vi "GetUserLayouts.vi"(8 "error in (no error)":errorcluster, 11 "Layout Ring Refnum":refnum<vi>) -> (0 "error out":errorcluster, 1 "Non-user Strings And Values []":T1, 2 "Value":i32, 3 "User StringsAndValues[]":T1, 4 "Num User Layouts":i32)   [LabVIEW 2013]
doc: "SetList table layouts consist of \"default\" layouts (ring val < 0) and user layouts (ring val >0). This VI separates the two, returning the input ring's \"Value\", \"User Strings and Values[]\" and \"Non-user layouts\" (also StringAndValue array)."
uses:
  <vilib>/Utility/miscctls.llb/LVStringsAndValuesArrayTypeDef_I32.ctl
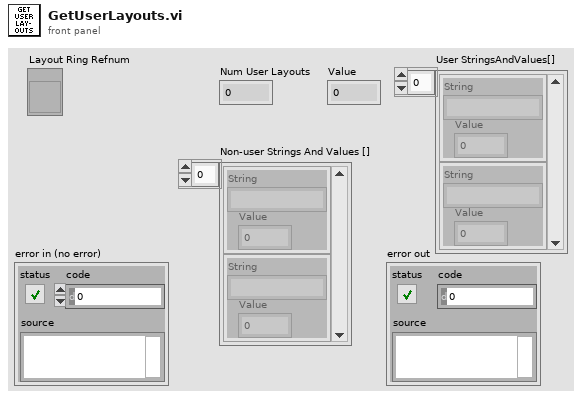
[diagram p1: front panel]
types:
  T1 = typedef "LVStringsAndValuesArrayTypeDef_I32.ctl" = cluster{"String":string, "Value":i32}[]
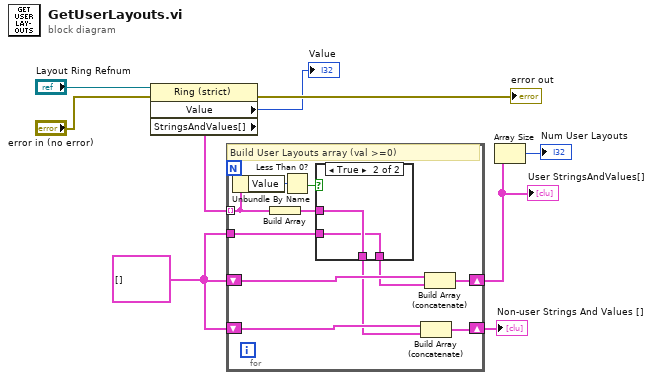
[diagram p0: block diagram]
diagram:
  w1 = T1 [] ("StringsAndValues[]")
  n1 = property class="Ring (strict)"(reference="Layout Ring Refnum", error in="error in (no error)") -> (error out=→"error out":errorcluster, "Value"=→"Value":i32, "StringsAndValues[]"=w2:T1)  [unwired: 1 out]
  n2 = for {
    tunnel: w2 -> [w10] mode=indexing
    shift-right: [w15] -> w4
    shift-left: w1 -> [w14]
    shift-right: [w16] -> w3
    shift-left: w1 -> [w17]
    tunnel: w1 -> [w18]
    # "Build User Layouts array (val >=0)"
    n3 = Unbundle By Name(w10) -> ("Value"=w20:i32)
    n4 = Build Array(w10) -> (w11:cluster{"String":string, "Value":i32}[])
    n5 = Less Than 0?(x=w20) -> (x < 0?=w19:bool)
    n6 = case shown="True" w19 {
      tunnel: w11 -> [w22 w24]
      tunnel: w18 -> [w21 w23]
      tunnel: [w21 w24] -> w13
      tunnel: [w22 w23] -> w12
      frame False {
      }
      frame True {
      }
    }
    n7 = Build Array (concatenate)(w17, w13) -> (w16:T1)
    n8 = Build Array (concatenate)(w14, w12) -> (w15:T1)
  }
  "User StringsAndValues[]" <- w4
  "Non-user Strings And Values []" <- w3
  n9 = Array Size(array=w4) -> (size(s)=→"Num User Layouts":i32)
